vi "Empty Data Check(IP).vi"(11 "element":T4) -> (3 "Empty?":bool)   [LabVIEW 2021]
uses:
  IP Simulation/Controls/IP_Cellular Tech Type def.ctl
  IP Simulation/Controls/IP_Network_Type def.ctl
  IP Simulation/Controls/IP_Type-Tydedef.ctl
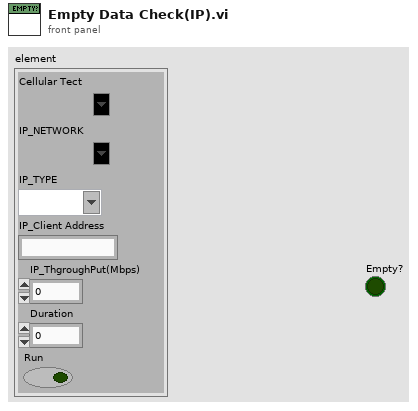
[diagram p1: front panel]
types:
  T1 = typedef "IP_Cellular Tech Type def.ctl" = string
  T2 = typedef "IP_Network_Type def.ctl" = string
  T3 = typedef "IP_Type-Tydedef.ctl" = string
  T4 = cluster{"Cellular Tect":T1, "IP_NETWORK":T2, "IP_TYPE":T3, "IP_Client Address":string, "IP_ThgroughPut(Mbps)":i32, "Duration":i32, "Run":bool}
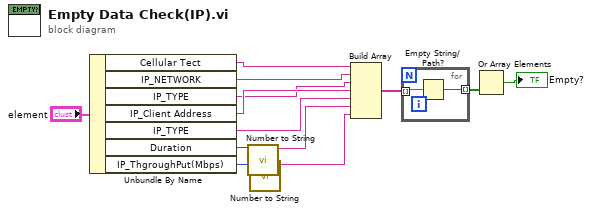
[diagram p0: block diagram]
diagram:
  n1 = Unbundle By Name("element") -> ("Cellular Tect"=w9:T1, "IP_NETWORK"=w10:T2, "IP_TYPE"=w11:T3, "IP_Client Address"=w12:string, "IP_TYPE"=w13:T3, "Duration"=w4:i32, "IP_ThgroughPut(Mbps)"=w3:i32)
  n2 = call "Number to String.vi"("DecimaL NU\nmber"=w4) -> ("Decimal String"=w2:string)  [unwired: 10 in]
  n3 = call "Number to String.vi"("DecimaL NU\nmber"=w3) -> ("Decimal String"=w1:string)  [unwired: 10 in]
  n4 = Build Array(w9, w10, w11, w12, w13, w2, w1) -> (w8:T3[])
  n5 = for {
    tunnel: w8 -> [w15] mode=indexing
    tunnel: [w14] -> w7 mode=indexing
    n6 = Empty String/Path?(string/path=w15) -> (empty?=w14:bool)
  }
  n7 = Or Array Elements(Boolean array=w7) -> (logical OR=→"Empty?":bool)
